vi "cluster_w_arrays2array.vi"(1 "BMS":T1={"Status"=0, "Vdc"=0.0, "Idc"=0.0, "SoC_max"=0.0, "SoC_min"=0.0, "SoH"=0, "SoCmods"=[0, 0, 0, 0, 0, 0, 0, 0, 0, 0, 0, 0, 0], "Tmods"=[0, 0, 0, 0, 0, 0, 0, 0, 0, 0, 0, 0, 0], "Warnings"=[], "Errors"=[], "Vcellmin"=[0.0, 0.0, 0.0, 0.0, 0.0, 0.0, 0.0, 0.0, 0.0, 0.0, 0.0, 0.0, 0.0], "Vcellmax"=[0.0, 0.0, 0.0, 0.0, 0.0, 0.0, 0.0, 0.0, 0.0, 0.0, 0.0, 0.0, 0.0], "Vmod"=[0.0, 0.0, 0.0, 0.0, 0.0, 0.0, 0.0, 0.0, 0.0, 0.0, 0.0, 0.0, 0.0]}) -> (0 "array":dbl[](array[numeric]))   [LabVIEW 2021]
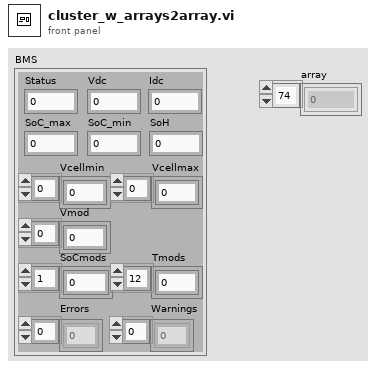
[diagram p1: front panel]
types:
  T1 = cluster{"Status":u16, "Vdc":dbl, "Idc":dbl, "SoC_max":dbl, "SoC_min":dbl, "SoH":u16, "SoCmods":u16[], "Tmods":u16[], "Warnings":u16[], "Errors":u16[], "Vcellmin":dbl[], "Vcellmax":dbl[], "Vmod":dbl[]}
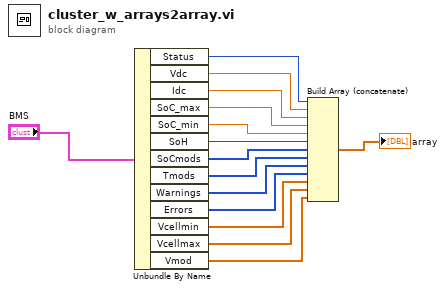
[diagram p0: block diagram]
diagram:
  n1 = Unbundle By Name("BMS") -> ("Status"=w15:u16, "Vdc"=w14:dbl, "Idc"=w13:dbl, "SoC_max"=w12:dbl, "SoC_min"=w11:dbl, "SoH"=w10:u16, "SoCmods"=w9:u16[], "Tmods"=w8:u16[], "Warnings"=w7:u16[], "Errors"=w6:u16[], "Vcellmin"=w5:dbl[], "Vcellmax"=w3:dbl[], "Vmod"=w2:dbl[])
  n2 = Build Array (concatenate)(w15, w14, w13, w12, w11, w10, w9, w8, w7, w6, w5, w3, w2) -> (→"array":dbl[])
